vi "Menu.Sequence.Load.vi"(8 "error in (no error)":errorcluster, 9 "Coords":T1, 10 "MenuRef":refnum<k9>, 11 "State Variables":T2={"Aliases.All"=[], "Aliases.Outputs"=[], "UI.Sequence#ofColumns"=0, "SysDef.Path"=path "", "UI.SequenceRef"=refnum, "UI.StepInformationRef"=refnum, "UI.AbortRef"=refnum, "UI.GraphRef"=refnum, "UI.ViewRef"=refnum, "UI.IterationsRef"=refnum, "UI.IterationInformationRef"=refnum, "INI.Settings"={"Build Location"=path "C:/Simple Sequence Editor/SequenceRepo", "LoggingLocation"=path ""}, "NIVS.Workspace Event"=refnum, "UI.SkipChannel"=refnum, "NIVS.Launched?"=FALSE, "UI.DurationChannel"=refnum}) -> (0 "error out":errorcluster, 3 "State Variables out":T2={"Aliases.All"=[], "Aliases.Outputs"=[], "UI.Sequence#ofColumns"=0, "SysDef.Path"=path "", "UI.SequenceRef"=refnum, "UI.StepInformationRef"=refnum, "UI.AbortRef"=refnum, "UI.GraphRef"=refnum, "UI.ViewRef"=refnum, "UI.IterationsRef"=refnum, "UI.IterationInformationRef"=refnum, "INI.Settings"={"Build Location"=path "C:/Simple Sequence Editor/SequenceRepo", "LoggingLocation"=path ""}, "NIVS.Workspace Event"=refnum, "UI.SkipChannel"=refnum, "NIVS.Launched?"=FALSE, "UI.DurationChannel"=refnum})   [LabVIEW 2013, in "Simple Sequence Tools - Editor.lvlib"]
uses:
  Simple Sequence Tools - Editor.lvlib
  Types/Main.StateVariables.ctl
  Shared/Types/Channel.Properties.ctl
  Shared/Types/INI.Settings
  <vilib>/Utility/miscctls.llb/LVPoint32TypeDef.ctl
  Shared/SubVIs/Main.Constants.vi
  Shared/Simple Sequence Tools - Shared.lvlib
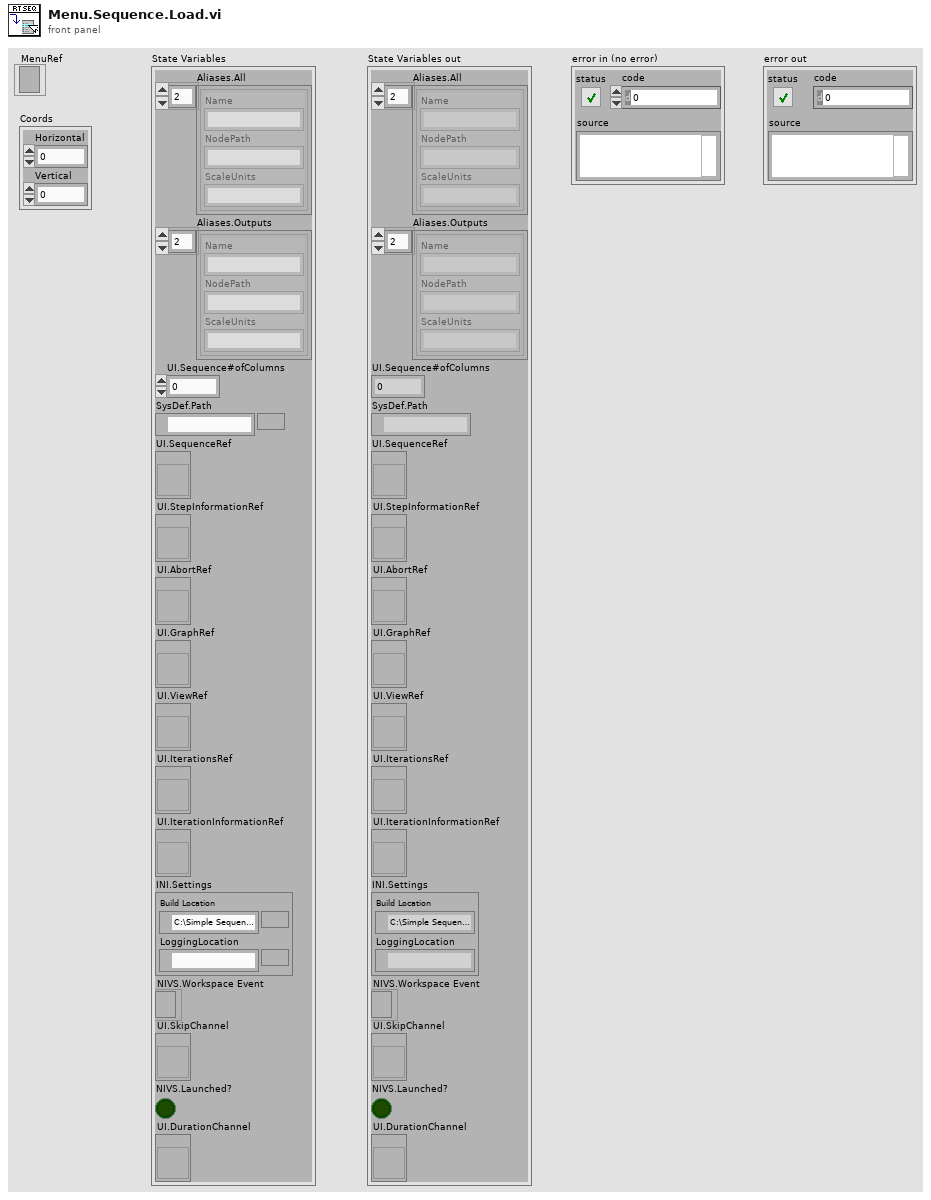
[diagram p1: front panel]
types:
  T1 = typedef "LVPoint32TypeDef.ctl" = cluster{"Horizontal":i32, "Vertical":i32}
  T2 = typedef "Simple Sequence Tools - Editor.lvlib/Main.StateVariables.ctl" = cluster{"Aliases.All":T3[], "Aliases.Outputs":T3[], "UI.Sequence#ofColumns":i32, "SysDef.Path":path, "UI.SequenceRef":refnum<vi>, "UI.StepInformationRef":refnum<vi>, "UI.AbortRef":refnum<vi>, "UI.GraphRef":refnum<vi>, "UI.ViewRef":refnum<vi>, "UI.IterationsRef":refnum<vi>, "UI.IterationInformationRef":refnum<vi>, "INI.Settings":T4, "NIVS.Workspace Event":refnum<event-registration>, "UI.SkipChannel":refnum<vi>, "NIVS.Launched?":bool, "UI.DurationChannel":refnum<vi>}
  T3 = typedef "Simple Sequence Tools - Shared.lvlib/Channel.Properties.ctl" = cluster{"Name":string, "NodePath":string, "ScaleUnits":string}
  T4 = typedef "Simple Sequence Tools - Shared.lvlib/INI.Settings" = cluster{"Build Location":path, "LoggingLocation":path}
  T5 = typedef "LVRowAndColumnTypeDef.ctl" = cluster{"Row":i32, "Column":i32}
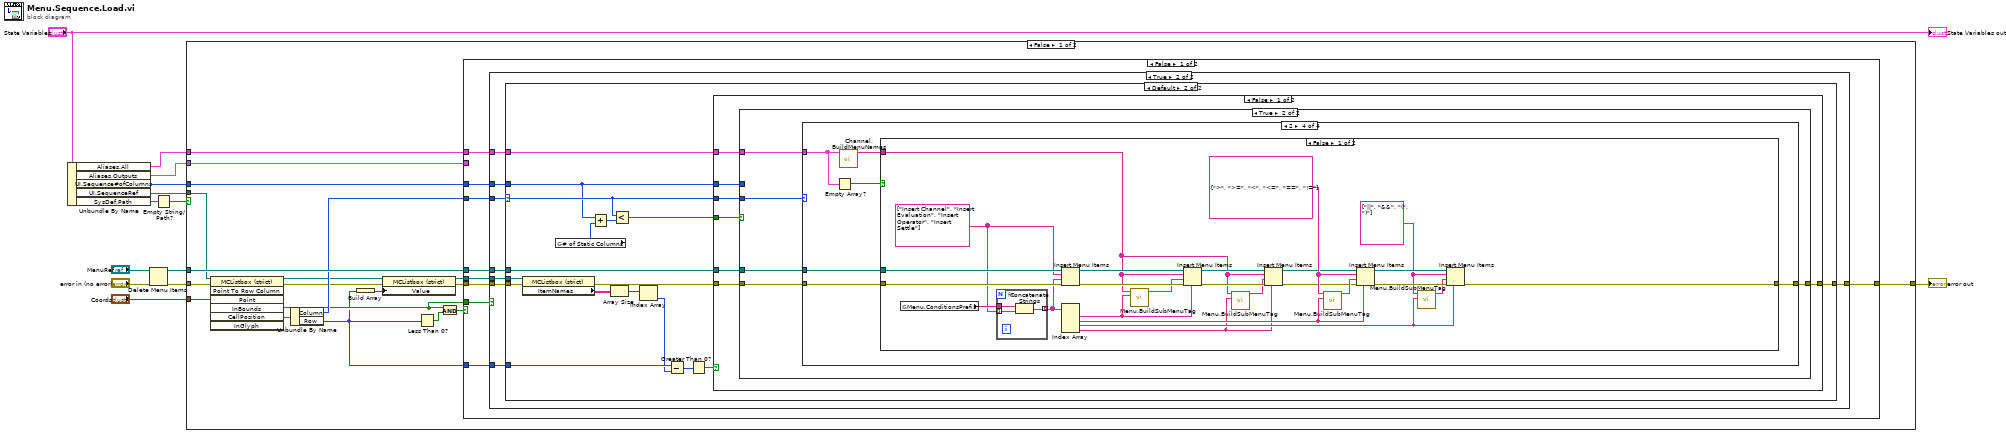
[diagram p0: block diagram]
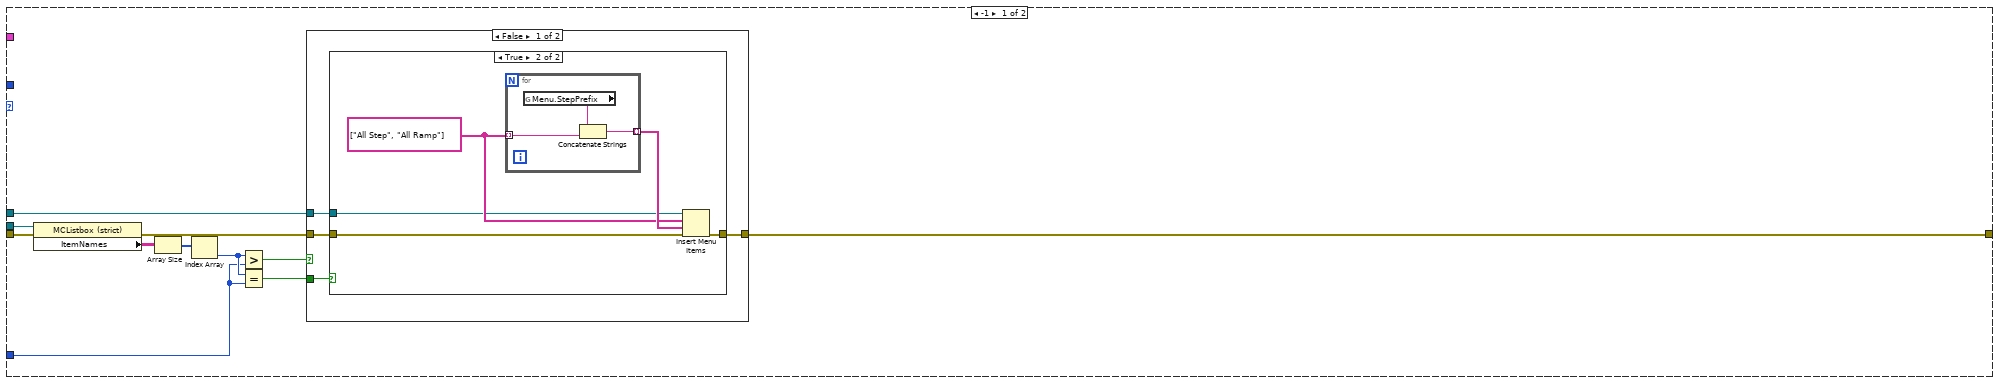
[diagram p3: hidden frame]
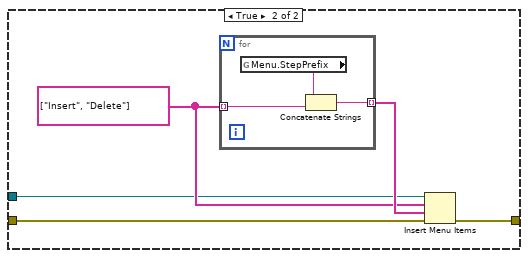
[diagram p5: hidden frame]
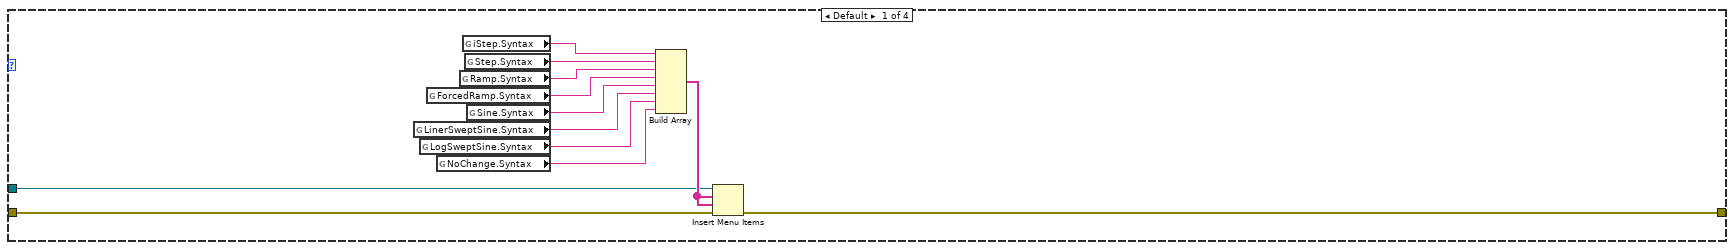
[diagram p7: hidden frame]
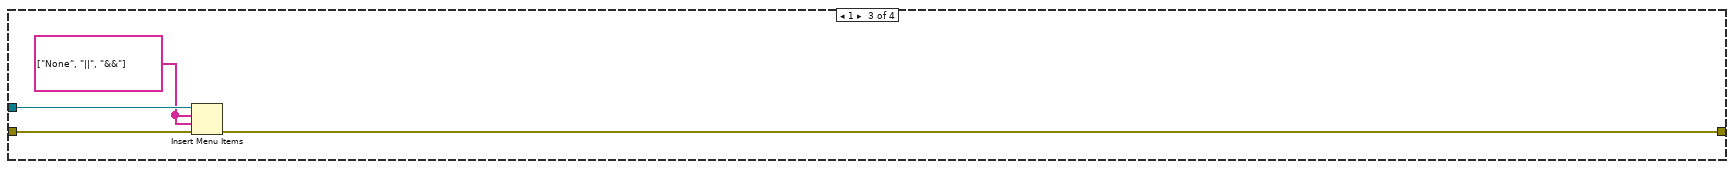
[diagram p9: hidden frame]
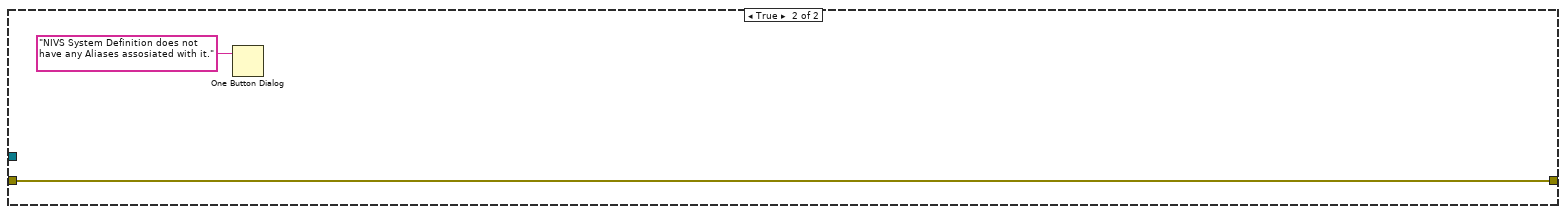
[diagram p10: hidden frame]
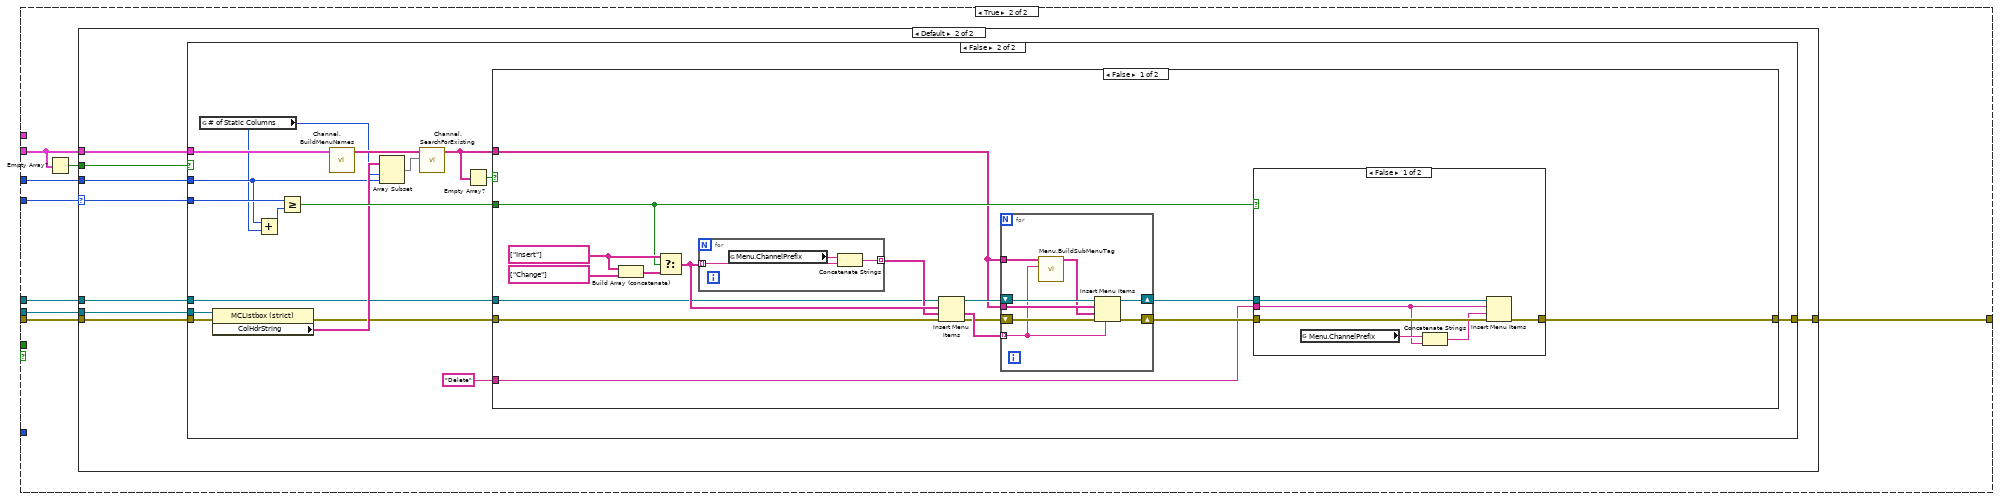
[diagram p12: hidden frame]
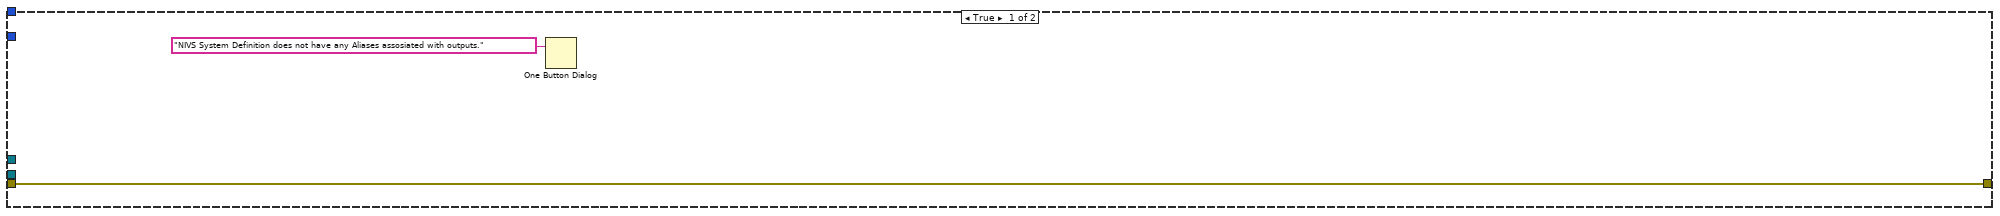
[diagram p14: hidden frame]
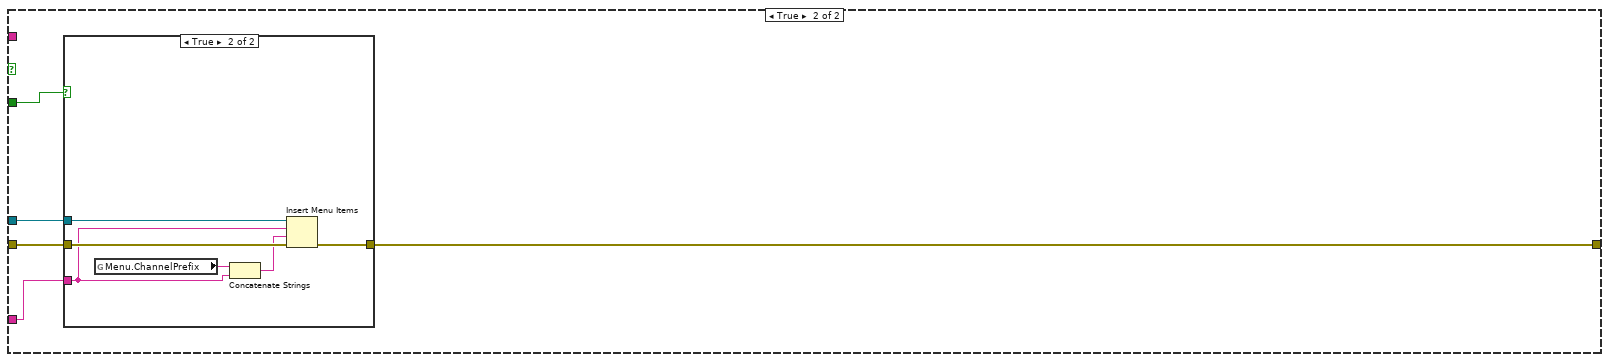
[diagram p16: hidden frame]
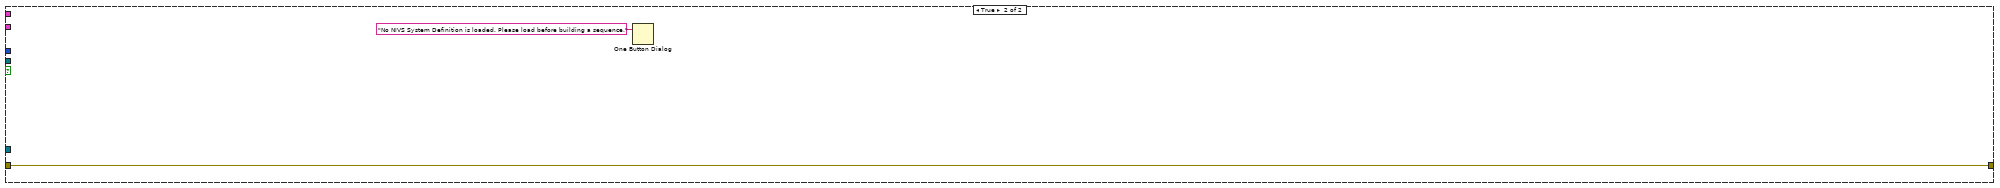
[diagram p18: hidden frame]
diagram:
  n1 = Unbundle By Name("State Variables") -> ("Aliases.All"=w1:T3[], "Aliases.Outputs"=w9:T3[], "UI.Sequence#ofColumns"=w12:i32, "UI.SequenceRef"=w10:refnum<vi>, "SysDef.Path"=w7:path)
  n2 = Delete Menu Items(6:"error in (no error)", 9:"MenuRef") -> (0:w4:errorcluster, 3:w2:refnum<k9>)  [unwired: 2 in]
  n3 = Empty String/Path?(string/path=w7) -> (empty?=w6:bool)
  n4 = case shown="False" w6 {
    tunnel: [w32 w249] -> w13
    tunnel: w2 -> [w31 _]
    tunnel: w12 -> [w30 _]
    tunnel: "Coords" -> [w25 _]
    tunnel: w10 -> [w24 _]
    tunnel: w4 -> [w23 w249]
    tunnel: w9 -> [w22 _]
    tunnel: w1 -> [w20 _]
    frame False {
      n5 = invoke class="MCListbox (strict)" method="Point To Row Column"(reference=w24, error in=w23, "Point"=w25) -> (reference out=w18:refnum<vi>, error out=w19:errorcluster, "InBounds"=w21:bool, "CellPosition"=w26:T5)  [unwired: 4 in, 3 out]
      n6 = Unbundle By Name(w26) -> ("Column"=w29:i32, "Row"=w15:i32)
      n7 = Build Array(w15) -> (w14:i32[])
      n8 = property class="MCListbox (strict)"(reference=w18, error in=w19, "Value"=w14) -> (reference out=w16:refnum<vi>, error out=w17:errorcluster)
      n9 = Less Than 0?(x=w15) -> (x < 0?=w27:bool)
      n10 = And(x=w21, y=w27) -> (x .and. y?=w28:bool)
      n11 = case shown="False" w28 {
        tunnel: w29 -> [w36 w167]
        tunnel: w30 -> [w37 w168]
        tunnel: w31 -> [w35 w171]
        tunnel: w17 -> [w40 w172]
        tunnel: [w34 w173] -> w32
        tunnel: w16 -> [w39 w174]
        tunnel: w22 -> [_ w170]
        tunnel: w21 -> [w41 _]
        tunnel: w15 -> [w38 _]
        tunnel: w20 -> [w33 _]
        frame False {
          n12 = case shown="True" w41 {
            tunnel: w40 -> [w42 w49]
            tunnel: w39 -> [_ w50]
            tunnel: w38 -> [_ w48]
            tunnel: w37 -> [_ w47]
            tunnel: w36 -> [_ w46]
            tunnel: w35 -> [_ w45]
            tunnel: [w42 w44] -> w34
            tunnel: w33 -> [_ w43]
            frame False {
            }
            frame True {
              n13 = case shown="Default" w46 {
                selector: w46 -> [_ w90]
                tunnel: w50 -> [w57 w99]
                tunnel: w49 -> [w59 w98]
                tunnel: w48 -> [w52 w95]
                tunnel: w47 -> [_ w84]
                tunnel: w45 -> [w60 w91]
                tunnel: [w61 w88] -> w44
                tunnel: w43 -> [_ w86]
                frame -1 {
                  n14 = property class="MCListbox (strict)"(reference=w57, error in=w59) -> (error out=w58:errorcluster, "ItemNames"=w55:string[][])  [unwired: 1 out]
                  n15 = Array Size(array=w55) -> (size(s)=w56:i32[])
                  n16 = Index Array(array=w56) -> (element=w53:i32)  [unwired: 1 in]
                  n17 = Greater?(x=w53, y=w52) -> (0:w54:bool)
                  n18 = Equal?(x=w53, y=w52) -> (x = y?=w51:bool)
                  n19 = case shown="False" w54 {
                    tunnel: [w64 w79] -> w61
                    tunnel: w60 -> [w63 w76]
                    tunnel: w58 -> [w65 w75]
                    tunnel: w51 -> [w62 _]
                    frame False {
                      n20 = case shown="True" w62 {
                        tunnel: w65 -> [w66 w69]
                        tunnel: [w66 w68] -> w64
                        tunnel: w63 -> [_ w67]
                        frame False {
                        }
                        frame True {
                          w70 = string[] ["All Step", "All Ramp"] ("item names")
                          n21 = for {
                            tunnel: [w73] -> w71 mode=indexing
                            tunnel: w70 -> [w74] mode=indexing
                            n22 = global read "Main.Constants.vi" "Menu.StepPrefix"() -> (w72:string)
                            n23 = Concatenate Strings(w72, w74) -> (w73:string)
                          }
                          n24 = Insert Menu Items(6:w69, 7:w71, 8:w70, 9:w67) -> (0:w68:errorcluster)  [unwired: 2 in, 2 out]
                        }
                      }
                    }
                    frame True {
                      w77 = string[] ["Insert", "Delete"] ("item names")
                      n25 = for {
                        tunnel: [w81] -> w78 mode=indexing
                        tunnel: w77 -> [w82] mode=indexing
                        n26 = global read "Main.Constants.vi" "Menu.StepPrefix"() -> (w80:string)
                        n27 = Concatenate Strings(w80, w82) -> (w81:string)
                      }
                      n28 = Insert Menu Items(6:w75, 7:w78, 8:w77, 9:w76) -> (0:w79:errorcluster)  [unwired: 2 in, 2 out]
                    }
                  }
                }
                frame Default {
                  n29 = property class="MCListbox (strict)"(reference=w99, error in=w98) -> (error out=w93:errorcluster, "ItemNames"=w97:string[][])  [unwired: 1 out]
                  n30 = global read "Main.Constants.vi" "# of Static Columns"() -> (w85:u32)
                  n31 = Add(x=w84, y=w85) -> (x+y=w83:u32)
                  n32 = Array Size(array=w97) -> (size(s)=w96:i32[])
                  n33 = Less?(x=w90, y=w83) -> (x < y?=w89:bool)
                  n34 = Index Array(array=w96) -> (element=w94:i32)  [unwired: 1 in]
                  n35 = Subtract(x=w95, y=w94) -> (x-y=w87:i32)
                  n36 = Greater Than 0?(x=w87) -> (x > 0?=w92:bool)
                  n37 = case shown="False" w92 {
                    tunnel: w93 -> [w106 w166]
                    tunnel: w84 -> [w103 _]
                    tunnel: w90 -> [w102 _]
                    tunnel: w91 -> [w105 _]
                    tunnel: w89 -> [w104 _]
                    tunnel: [w101 w166] -> w88
                    tunnel: w86 -> [w100 _]
                    frame False {
                      n38 = case shown="True" w104 {
                        tunnel: w106 -> [w107 w111]
                        tunnel: w105 -> [_ w112]
                        tunnel: w103 -> [_ _]
                        tunnel: w102 -> [_ w108]
                        tunnel: [w107 w110] -> w101
                        tunnel: w100 -> [_ w109]
                        frame False {
                        }
                        frame True {
                          n39 = case shown="2" w108 {
                            tunnel: w112 -> [w113 _ w129 w135]
                            tunnel: w111 -> [w115 w125 w128 w134]
                            tunnel: [w114 w125 w126 w133] -> w110
                            tunnel: w109 -> [_ _ _ w132]
                            frame Default {
                              n40 = global read "Main.Constants.vi" "LinerSweptSine.Syntax"() -> (w119:string)
                              n41 = global read "Main.Constants.vi" "LogSweptSine.Syntax"() -> (w116:string)
                              n42 = global read "Main.Constants.vi" "ForcedRamp.Syntax"() -> (w117:string)
                              n43 = global read "Main.Constants.vi" "NoChange.Syntax"() -> (w122:string)
                              n44 = global read "Main.Constants.vi" "Ramp.Syntax"() -> (w118:string)
                              n45 = global read "Main.Constants.vi" "iStep.Syntax"() -> (w121:string)
                              n46 = global read "Main.Constants.vi" "Step.Syntax"() -> (w124:string)
                              n47 = global read "Main.Constants.vi" "Sine.Syntax"() -> (w120:string)
                              n48 = Build Array(w121, w124, w118, w117, w120, w119, w116, w122) -> (w123:string[])
                              n49 = Insert Menu Items(6:w115, 7:w123, 8:w123, 9:w113) -> (0:w114:errorcluster)  [unwired: 2 in, 2 out]
                            }
                            frame 0 {
                            }
                            frame 1 {
                              w127 = string[] ["None", "||", "&&"] ("item names")
                              n50 = Insert Menu Items(6:w128, 7:w127, 8:w127, 9:w129) -> (0:w126:errorcluster)  [unwired: 2 in, 2 out]
                            }
                            frame 2 {
                              n51 = Empty Array?(array=w132) -> (empty?=w131:bool)
                              n52 = call "Channel.BuildMenuNames.vi"("Aliases"=w132) -> ("Aliases Array"=w130:string[])  [unwired: 10 in]
                              n53 = case shown="False" w131 {
                                tunnel: w135 -> [w160 _]
                                tunnel: w134 -> [w159 w164]
                                tunnel: [w144 w164] -> w133
                                tunnel: w130 -> [w137 _]
                                frame False {
                                w146 = string[] [">", ">=", "<", "<=", "==", "!="] ("item names")
                                w145 = string[] ["||", "&&", "(", ")"] ("item names")
                                w157 = string[] ["Insert Channel", "Insert Evaluation", "Insert Operator", "Insert Settle"] ("item names")
                                n54 = global read "Main.Constants.vi" "Menu.ConditionsPrefix"() -> (w158:string)
                                n55 = for {
                                tunnel: w157 -> [w163] mode=indexing
                                tunnel: w158 -> [w162]
                                tunnel: [w161] -> w153 mode=indexing
                                n56 = Concatenate Strings(w162, w163) -> (w161:string)
                                }
                                n57 = Insert Menu Items(6:w159, 7:w153, 8:w157, 9:w160) -> (0:w156:errorcluster, 3:w155:refnum<k9>)  [unwired: 2 in, 1 out]
                                n58 = Index Array(array=w153) -> (element #1=w154:string, element #2=w150:string, element #3=w148:string, element #4=w136:string)  [unwired: 4 in]
                                n59 = call "Menu.BuildSubMenuTag.vi"("Menu"=w154, "Aliases Array"=w137) -> ("Tag Array"=w139:string[])  [unwired: 9 in]
                                n60 = Insert Menu Items(5:w154, 6:w156, 7:w139, 8:w137, 9:w155) -> (0:w143:errorcluster, 3:w141:refnum<k9>)  [unwired: 1 in, 1 out]
                                n61 = call "Menu.BuildSubMenuTag.vi"("Menu"=w136, "Aliases Array"=w137) -> ("Tag Array"=w138:string[])  [unwired: 9 in]
                                n62 = Insert Menu Items(5:w136, 6:w143, 7:w138, 8:w137, 9:w141) -> (0:w142:errorcluster, 3:w140:refnum<k9>)  [unwired: 1 in, 1 out]
                                n63 = call "Menu.BuildSubMenuTag.vi"("Menu"=w150, "Aliases Array"=w146) -> ("Tag Array"=w149:string[])  [unwired: 9 in]
                                n64 = Insert Menu Items(5:w150, 6:w142, 7:w149, 8:w146, 9:w140) -> (0:w152:errorcluster, 3:w151:refnum<k9>)  [unwired: 1 in, 1 out]
                                n65 = call "Menu.BuildSubMenuTag.vi"("Menu"=w148, "Aliases Array"=w145) -> ("Tag Array"=w147:string[])  [unwired: 9 in]
                                n66 = Insert Menu Items(5:w148, 6:w152, 7:w147, 8:w145, 9:w151) -> (0:w144:errorcluster)  [unwired: 1 in, 2 out]
                                }
                                frame True {
                                n67 = One Button Dialog(message="NIVS System Definition does not have any Aliases assosiated with it.") -> ()  [unwired: 1 in, 1 out]
                                }
                              }
                            }
                          }
                        }
                      }
                    }
                    frame True {
                    }
                  }
                }
              }
            }
          }
        }
        frame True {
          n68 = Empty Array?(array=w170) -> (empty?=w169:bool)
          n69 = case shown="Default" w167 {
            selector: w167 -> [_ w176]
            tunnel: w174 -> [_ w183]
            tunnel: [w175 w182] -> w173
            tunnel: w172 -> [w175 w181]
            tunnel: w171 -> [_ w180]
            tunnel: w170 -> [_ w179]
            tunnel: w169 -> [_ w178]
            tunnel: w168 -> [_ w177]
            frame -1..2 {
            }
            frame Default {
              n70 = case shown="False" w178 {
                tunnel: w176 -> [_ w189]
                tunnel: w183 -> [_ w201]
                tunnel: w177 -> [_ w188]
                tunnel: [w185 w199] -> w182
                tunnel: w179 -> [_ w198]
                tunnel: w181 -> [w185 w194]
                tunnel: w180 -> [_ w195]
                frame True {
                  n71 = One Button Dialog(message="NIVS System Definition does not have any Aliases assosiated with outputs.") -> ()  [unwired: 1 in, 1 out]
                }
                frame False {
                  n72 = global read "Main.Constants.vi" "# of Static Columns"() -> (w187:u32)
                  n73 = property class="MCListbox (strict)"(reference=w201, error in=w194) -> (error out=w193:errorcluster, "ColHdrString"=w200:string[])  [unwired: 1 out]
                  n74 = Add(x=w188, y=w187) -> (x+y=w186:u32)
                  n75 = Greater Or Equal?(x=w189, y=w186) -> (x >= y?=w202:bool)
                  n76 = call "Channel.BuildMenuNames.vi"("Aliases"=w198) -> ("Aliases Array"=w196:string[])  [unwired: 10 in]
                  n77 = Array Subset(array=w200, index=w187, length=w188) -> (w197:string[])
                  n78 = call "Channel.SearchForExisting.vi"("Existing Channels"=w197, "All Channels"=w196) -> ("Array out"=w192:string[])  [unwired: 9 in]
                  n79 = Empty Array?(array=w192) -> (empty?=w191:bool)
                  n80 = case shown="False" w191 {
                    tunnel: w202 -> [w204 w237]
                    tunnel: [w207 w240] -> w199
                    tunnel: w195 -> [w211 w239]
                    tunnel: w192 -> [w203 _]
                    tunnel: w193 -> [w209 w241]
                    tunnel: "Delete" ("string") -> [w205 w238]
                    frame False {
                      w216 = string[] ["Insert"]
                      n81 = Build Array (concatenate)(w216, string[] ["Change"]) -> (w217:string[])
                      n82 = Select(t=w216, s=w204, f=w217) -> (s? t:f=w215:string[])
                      n83 = for {
                        tunnel: w215 -> [w236] mode=indexing
                        tunnel: [w235] -> w214 mode=indexing
                        n84 = global read "Main.Constants.vi" "Menu.ChannelPrefix"() -> (w234:string)
                        n85 = Concatenate Strings(w234, w236) -> (w235:string)
                      }
                      n86 = Insert Menu Items(6:w209, 7:w214, 8:w215, 9:w211) -> (0:w210:errorcluster, 1:w212:string[], 3:w213:refnum<k9>)  [unwired: 2 in]
                      n87 = for {
                        tunnel: w212 -> [w228] mode=indexing
                        shift-right: [w232] -> w208
                        shift-left: w210 -> [w233]
                        tunnel: w203 -> [w230]
                        shift-right: [w229] -> w206
                        shift-left: w213 -> [w231]
                        tunnel: w203 -> [w227]
                        n88 = call "Menu.BuildSubMenuTag.vi"("Menu"=w228, "Aliases Array"=w227) -> ("Tag Array"=w226:string[])  [unwired: 9 in]
                        n89 = Insert Menu Items(5:w228, 6:w233, 7:w226, 8:w230, 9:w231) -> (0:w232:errorcluster, 3:w229:refnum<k9>)  [unwired: 1 in, 1 out]
                      }
                      n90 = case shown="False" w204 {
                        tunnel: w208 -> [w224 w225]
                        tunnel: [w223 w225] -> w207
                        tunnel: w206 -> [w222 _]
                        tunnel: w205 -> [w219 _]
                        frame False {
                          n91 = global read "Main.Constants.vi" "Menu.ChannelPrefix"() -> (w221:string)
                          n92 = Concatenate Strings(w221, w219) -> (w220:string)
                          n93 = Insert Menu Items(6:w224, 7:w220, 8:w219, 9:w222) -> (0:w223:errorcluster)  [unwired: 2 in, 2 out]
                        }
                        frame True {
                        }
                      }
                    }
                    frame True {
                      n94 = case shown="True" w237 {
                        tunnel: w241 -> [w242 w248]
                        tunnel: [w242 w247] -> w240
                        tunnel: w239 -> [_ w246]
                        tunnel: w238 -> [_ w244]
                        frame False {
                        }
                        frame True {
                          n95 = global read "Main.Constants.vi" "Menu.ChannelPrefix"() -> (w245:string)
                          n96 = Concatenate Strings(w245, w244) -> (w243:string)
                          n97 = Insert Menu Items(6:w248, 7:w243, 8:w244, 9:w246) -> (0:w247:errorcluster)  [unwired: 2 in, 2 out]
                        }
                      }
                    }
                  }
                }
              }
            }
          }
        }
      }
    }
    frame True {
      n98 = One Button Dialog(message="No NIVS System Definition is loaded. Please load before building a sequence.") -> ()  [unwired: 1 in, 1 out]
    }
  }
  "error out" <- w13
  "State Variables out" <- "State Variables"
